vi "Motion Profile Tester.vi"() -> ()   [LabVIEW 2015]
uses:
  <vilib>/Rock Robotics/WPI/CAN/TalonSRX/WPI_CANTalonSRX_APIFeedbackSelect.ctl
  <vilib>/Rock Robotics/WPI/CAN/TalonSRX/WPI_CANTalonSRX_MotionProfileTrajectoryPt.ctl
  <vilib>/Rock Robotics/WPI/CAN/TalonSRX/WPI_CANTalonSRX_APIControlMode.ctl
  <vilib>/Rock Robotics/WPI/MotorControl/WPI_MotorControlOpenCANTalonSRX.vi
panel:
  in  "Slave Motor Inverts":bool[](array[boolean])
  in  "Motor ID":dbl
  in  "Slave Motor IDs":dbl[](array[numeric])
  out "Current State":T1(ring)
  in  "Invert Motor":bool=TRUE
  in  "Execute Motion Profile using only Feedfoward":bool
  in  "Soft Limits (rotations)":T2={"Forward Limit Position"=10000.0, "Reverse Limit Position (should be less than foward limit position)"=-10000.0}
  in  "Reverse Soft Limit Enable":bool
  in  "Forward Soft Limit Enable":bool
  in  "Reverse Feedback Sensor":bool
  in  "Feedback Reference":T3=enum."CTR Magnetic Enc (Absolute)"
  in  "PID Values":T4={"P"=0.21, "I"=0.0021, "D"=3.0, "F"=0.12, "I Zone"=1200.0}
  out "error out":errorcluster
  out "Motor Values while Running Profile":cluster{dbl[], dbl[]}[](graph)
  out "Applied Throttle while Running Profile":cluster{dbl[], dbl[]}(graph)
  in  "Run at 100% Power and Graph":bool
  in  "Abort":bool
  in  "Generate, Load, and Run Profile":bool
  in  "Run Profile":bool
  in  "Load Profile":bool
  in  "Generate Profile and Clear Points":bool
  out "Generated Profile":cluster{dbl[], dbl[]}[](graph)
  in  "Mode":T1(ring)
  in  "Motion Profile Control Frame Rate":dbl=10.0
  in  "Rotations to Travel":dbl
  in  "Max Jerk (rotations/sec^3)":dbl
  in  "Max Acceleration (rotations/sec^2)":dbl
  in  "Max Speed (rotations/sec)":dbl
  # "Basic Motor Configuration Settings"
  # "Motion Profile Settings"
  # "If applied throttle exceeds about .95 at any point in the execution of the profile either max speed acceleration, or jerk must be lowered (or PIDF should be adjusted). If it goes below .8 except at the very beginning or end either max speed, acceleration, or jerk  could be increased. (These numbers are for profiles which are supposed to be completed as quickly as possible. In contexts where the priority is on other things such as reducing the amount of force or jerk acting on a gearbox other metrics must be used.)"
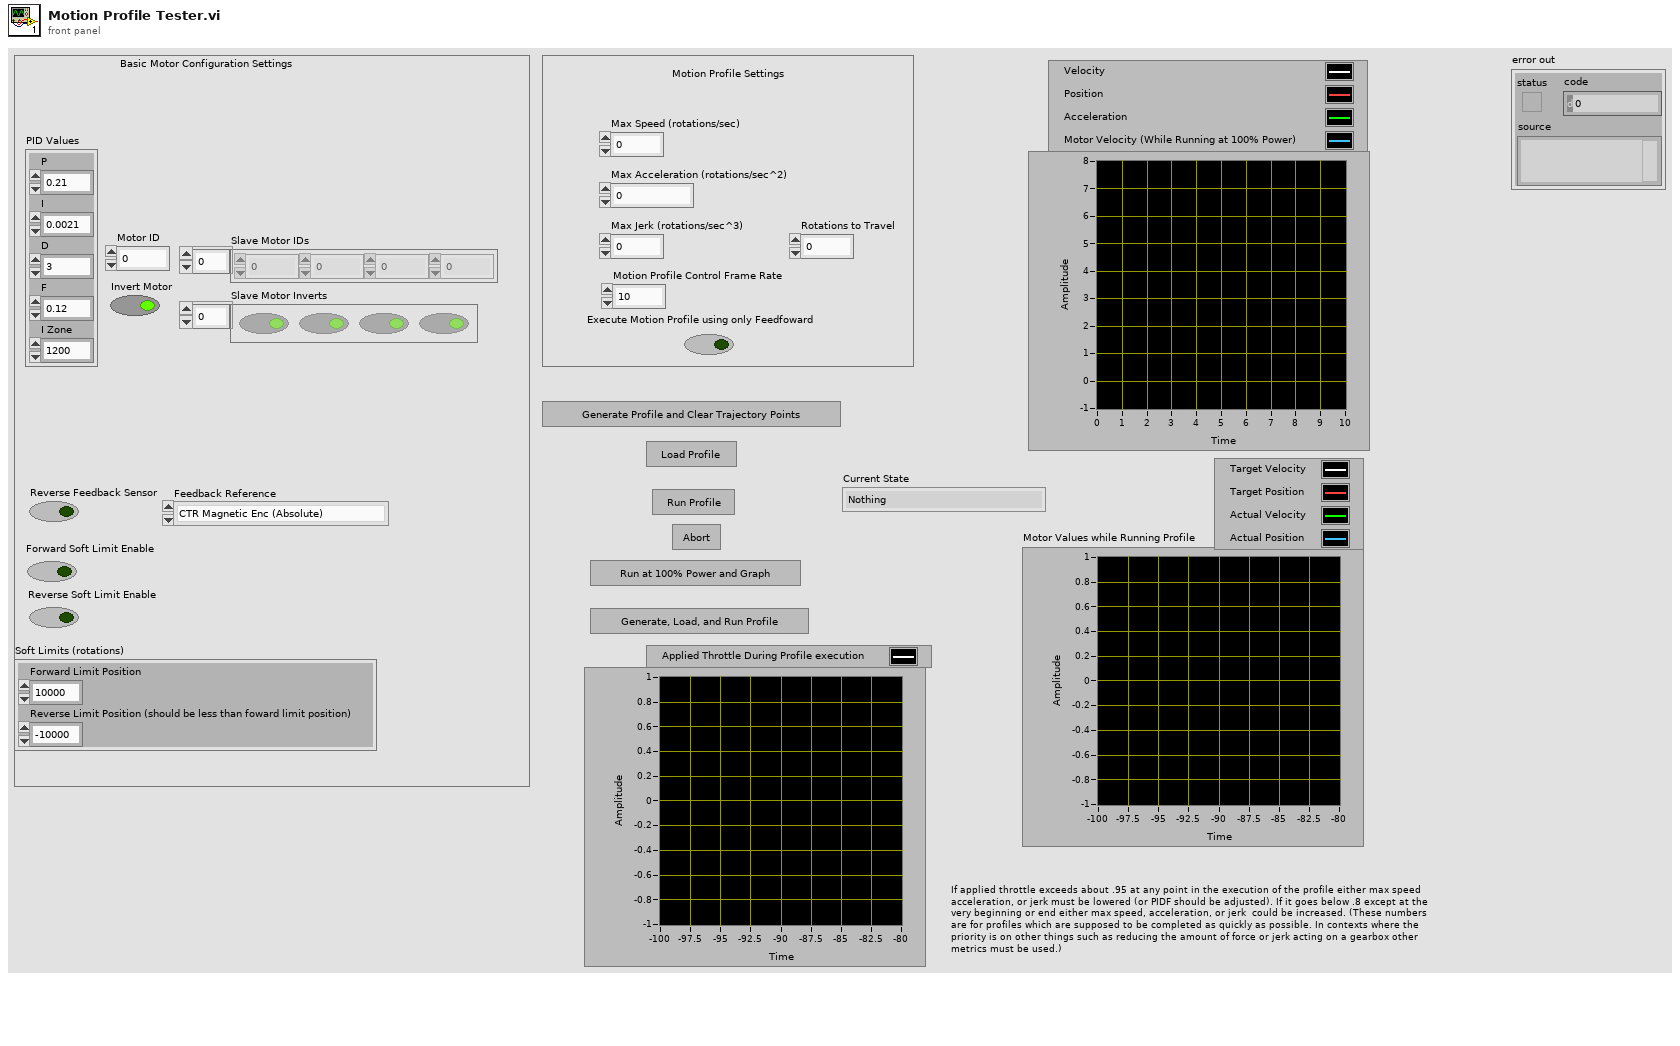
[diagram p1: front panel]
types:
  T1 = enum16{"Nothing", "Generate Profile and Clear", "Load Data to Motor", "Run Profile", "Run at 100% power and log"}
  T2 = cluster{"Forward Limit Position":dbl, "Reverse Limit Position (should be less than foward limit position)":dbl}
  T3 = typedef "WPI_CANTalonSRX_APIFeedbackSelect.ctl" = enum16{"Digital Quadrature Encoder", "Analog Potentiometer", "Analog Encoder", "Count on Quad-A (Rising-Edge)", "Count on Quad-A (Falling-Edge)", "CTR Magnetic Enc (Absolute)", "CTR Magnetic Enc (Relative)", "Pulse Width"}
  T4 = cluster{"P":dbl, "I":dbl, "D":dbl, "F":dbl, "I Zone":dbl}
  T5 = typedef "WPI_CANTalonSRX_APIControlMode.ctl" = enum8{"Percent VBus", "Speed", "Position", "Slave", "Unchanged / Invalid", "Voltage Compensation", "Current", "Motion Profile"}
  T6 = typedef "WPI_MotorControlDeviceRef.ctl" = cluster{"DeviceStatus":errorcluster, "Type":T7, "PWM":cluster{"PWM Channel":T8, "DeadBand":T9}, "CAN":cluster{"Device Number":u8, "Control Mode":T10, "Semaphore":T11, "Max Vout":dbl, "TalonSRX Control Mode":T5}, "Invert":bool}
  T7 = typedef "WPI_MotorControlType.ctl" = enum16{"PWM", "CAN", "CANTalonSRX"}
  T8 = typedef "FPGA_DIOPWMChannel.ctl" = enum8{"PWM 0", "PWM 1", "PWM 2", "PWM 3", "PWM 4", "PWM 5", "PWM 6", "PWM 7", "PWM 8", "PWM 9", "PWM MXP 0", "PWM MXP 1", "PWM MXP 2", "PWM MXP 3", "PWM MXP 4", "PWM MXP 5", "PWM MXP 6", "PWM MXP 7", "PWM MXP 8", "PWM MXP 9", "Invalid"}
  T9 = typedef "WPI_PWMDeadband.ctl" = cluster{"Name":string, "maxPositivePwm":i32, "minPositivePwm":i32, "centerPwm":i32, "maxNegativePwm":i32, "minNegativePwm":i32, "angularRange":u16}
  T10 = typedef "WPI_CANJaguar_ControlMode.ctl" = enum8{"Percent VBus", "Current", "Speed", "Position", "Voltage"}
  T11 = typedef "Semaphore RefNum" = refnum<k1>
  T12 = typedef "WPI_CANTalonSRX_MotionProfileTrajectoryPt.ctl" = cluster{"Duration Ms":u8, "Velocity":dbl, "Position":dbl, "Profile Slot Select":u8, "Is Last":bool, "Velocity Only":bool, "Zero Position":bool, "Compress Code":u8, "Same Velocity":i32, "Delta Position":i32, "Count":u8}
  T13 = enum16{"Nothing", "Generate Profile and Clear", "Load Data to Motor", "Run Profile"}
  T14 = enum16{"Nothing", "Generate Profile and Clear", "Load Data to Motor", "Run Profile", "Run at 100% power and log"}[]
  T15 = typedef "WPI_CANTalonSRX_GlobalStatus.ctl" = cluster{"Applied Throttle":dbl, "Module Enabled":bool, "CAN Error":errorcluster, "Closed Loop Error":dbl, "Forward Limit Switch Closed":bool, "Reverse Limit Switch Closed":bool, "Sensor Position":dbl, "Sensor Velocity":dbl, "Current":dbl, "Sticky Fault - Over Temp":bool, "Sticky Fault - Under Voltage":bool, "Sticky Fault - Forward Limit":bool, "Sticky Fault - Reverse Limit":bool, "Sticky Fault - Forward Soft Limit":bool, "Sticky Fault - Reverse Soft Limit":bool, "Brake is Enabled":bool, "Encoder Position":dbl, "Encoder Velocity":dbl, "Encoder Index Count":dbl, "Encoder A Pin State":bool, "Encoder B Pin State":bool, "Encoder Index Pin State":bool, "Analog In":dbl, "Analog In Velocity":dbl, "Temperature (C)":dbl, "Battery Voltage":dbl, "Control 5 Is Supported":bool, "Current Profile Slot Select":dbl, "Pos Div 8":bool, "Vel Div 4":bool, "Pulse Width Position":i32, "Pulse Width Velocity":i32, "Pulse Width Rise To Rise (us)":i32, "Pulse Width Rise To Fall (us)":i32, "Mot Prof Active Is Under Run":bool, "Mot Prof Active Has Under Run":bool, "Mot Prof Active Is Last":bool, "Mot Prof Active Velocity Only":bool, "Mot Prof Active Is Valid":bool, "Mot Prof Buffer Is Full":bool, "Mot Prof Active Profile Slot Select":i32, "Mot Prof NextID":i32, "Mot Prof Count":i32, "Mot Prof Active Velocity":dbl, "Mot Prof Active Position":dbl, "Mot Prof Output Enable":i32}
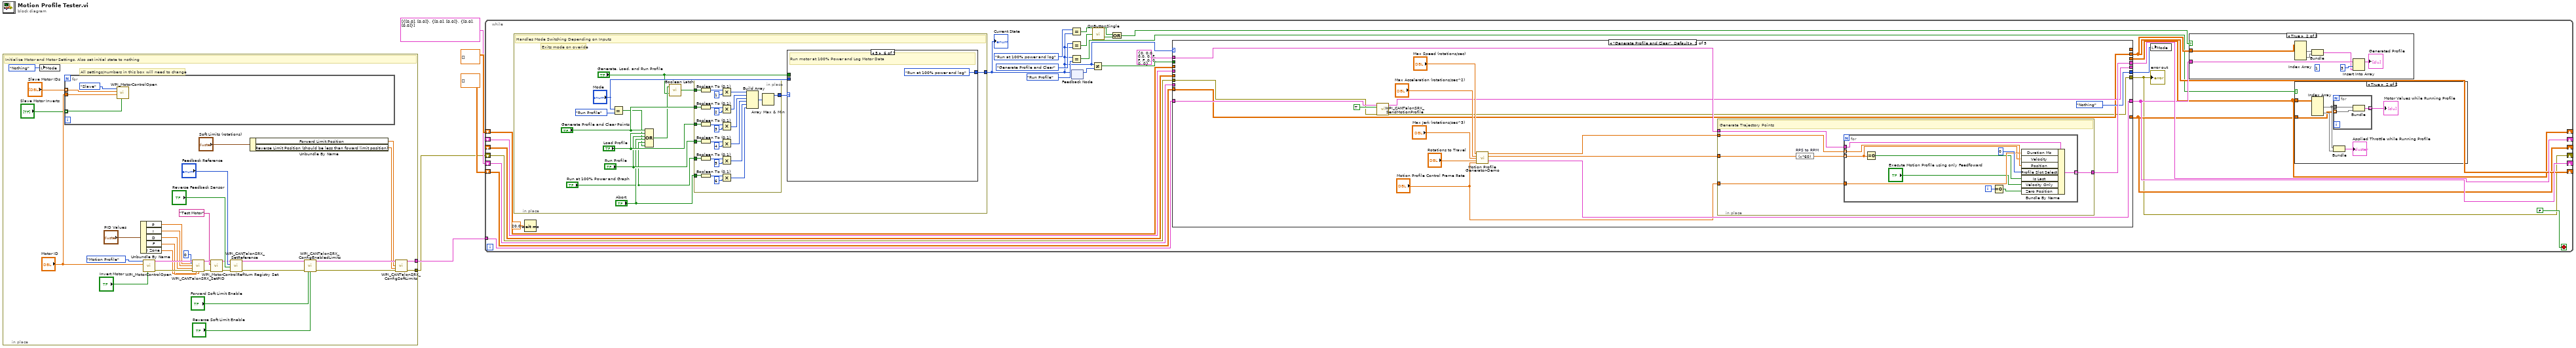
[diagram p0: block diagram]
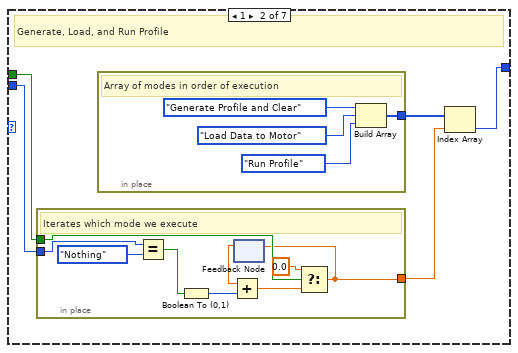
[diagram p5: hidden frame]
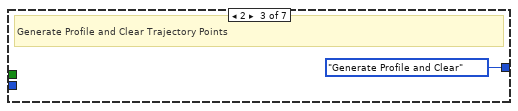
[diagram p6: hidden frame]
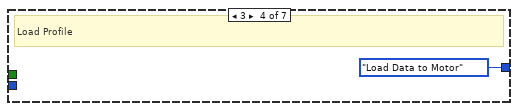
[diagram p7: hidden frame]
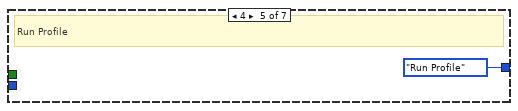
[diagram p8: hidden frame]
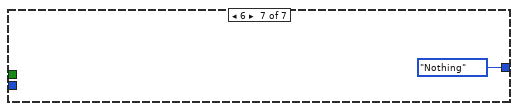
[diagram p9: hidden frame]
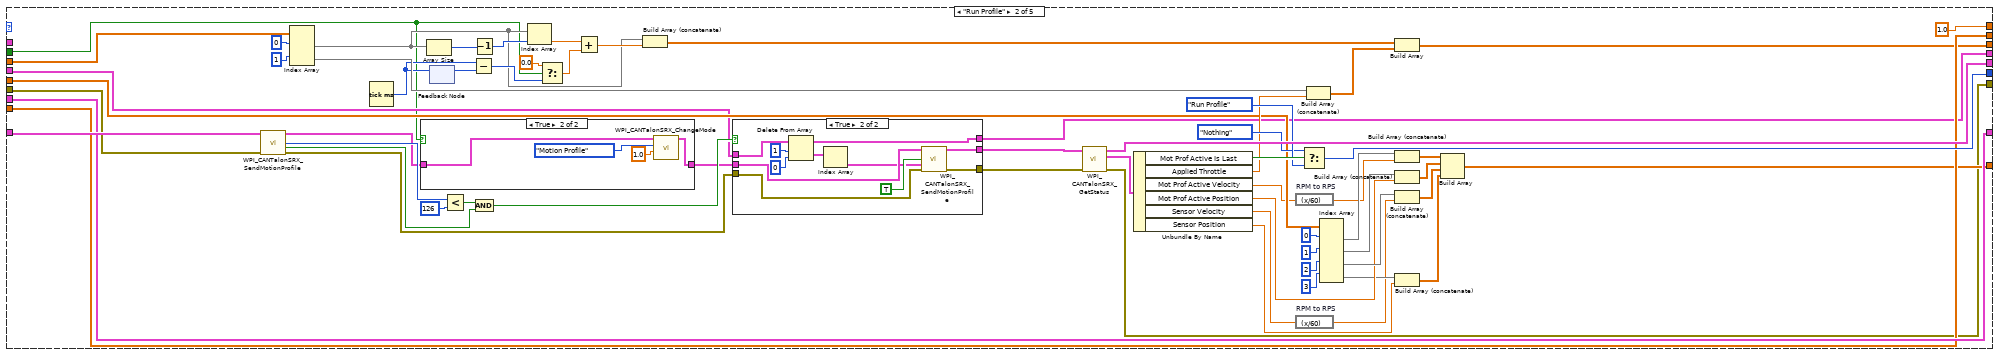
[diagram p10: hidden frame]
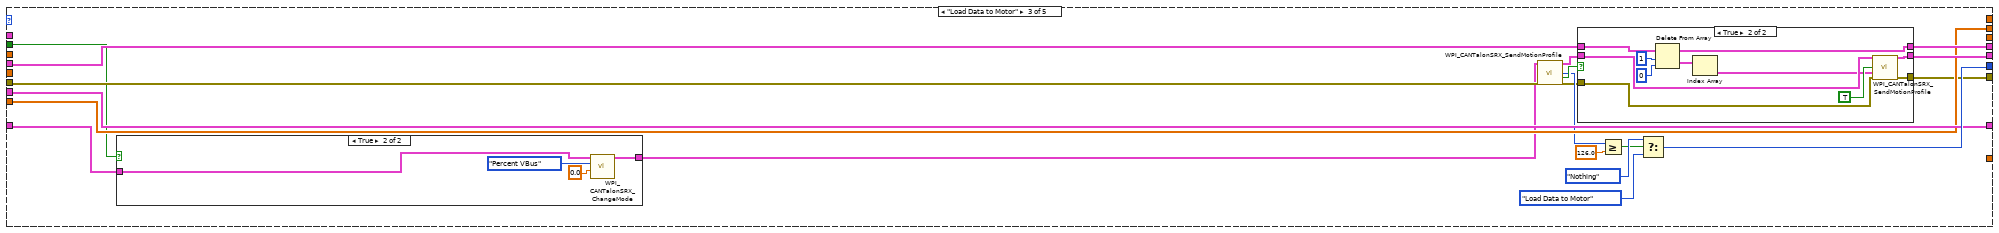
[diagram p13: hidden frame]
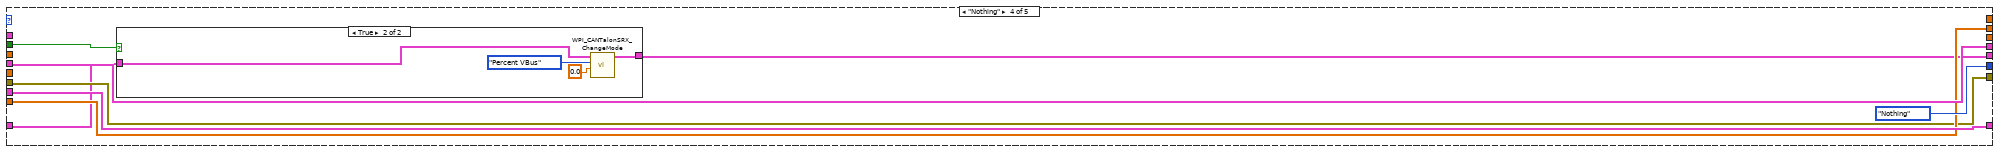
[diagram p16: hidden frame]
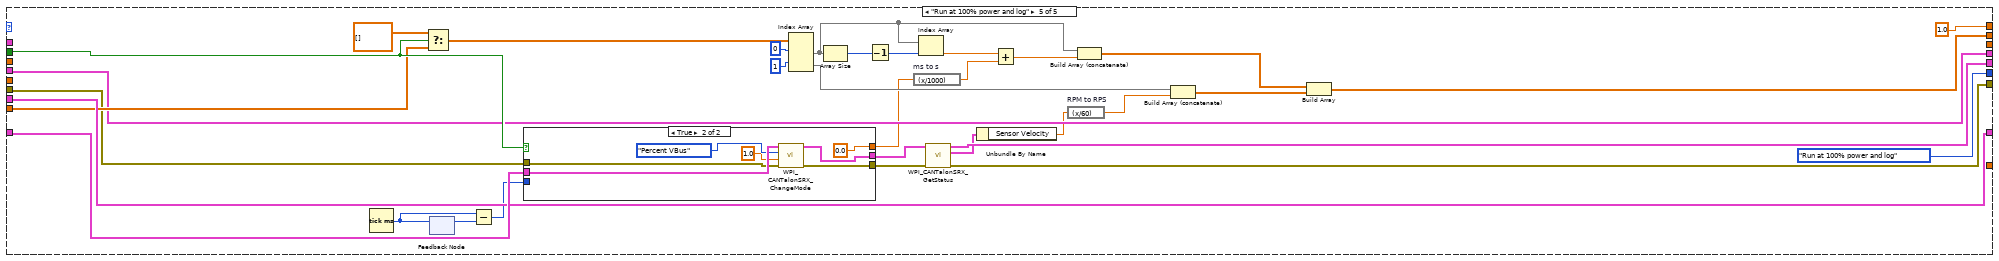
[diagram p18: hidden frame]
diagram:
  n1 = in-place {
    in-place-border: [w33] -> w5
    in-place-border: [w20] -> w1
    # "All settings/numbers in this box will need to change"
    # "Initialize Motor and Motor Settings. Also set initial state to nothing"
    n2 = local write "Mode"(T1."Nothing" ("Mode")) -> ()
    n3 = for {
      tunnel: "Motor ID" -> [w42]
      tunnel: "Slave Motor IDs" -> [w41] mode=indexing
      tunnel: "Slave Motor Inverts" -> [w39] mode=indexing
      n4 = call-poly <vilib>:"WPI_MotorControlOpen.vi"("Invert"=w39, "Master Device Number"=w42, "Device Number"=w41, "Control Mode"=WPI_CANTalonSRX_APIControlMode."Slave") -> ()  [unwired: 6 in, 2 out]
    }
    n5 = Unbundle By Name("PID Values") -> ("P"=w13:dbl, "I"=w12:dbl, "D"=w11:dbl, "F"=w10:dbl, "I Zone"=w9:dbl)
    n6 = call-poly <vilib>:"WPI_MotorControlOpen.vi"("Invert"="Invert Motor", "Device Number"="Motor ID", "Control Mode"=WPI_CANTalonSRX_APIControlMode."Motion Profile") -> ("error out"=w36:errorcluster, "MotorControlDeviceRef"=w37:T6)  [unwired: 7 in]
    n7 = call <vilib>:"WPI_CANTalonSRX_SetPID.vi"("CAN Talon SRX Ref"=w37, "Parameter Slot"=u8 0, "P"=w13, "I"=w12, "D"=w11, "error in (no error)"=w36, "F"=w10, "I Zone"=w9) -> ("CAN Talon SRX Ref"=w28:T6, "error out"=w26:errorcluster)  [unwired: 6 in]
    n8 = call <vilib>:"WPI_MotorControlRefNum Registry Set.vi"("error in (no error)"=w26, "refnum name"="Test Motor", "MotorControlDevRef"=w28) -> ("error out"=w25:errorcluster, "MotorControlDevRef"=w27:T6)  [unwired: 7 in]
    n9 = call <vilib>:"WPI_CANTalonSRX_SetReference.vi"("error in (no error)"=w25, "Reverse Feedback Sensor"="Reverse Feedback Sensor", "Feedback Reference"="Feedback Reference", "CAN Talon SRX Ref"=w27) -> ("error out"=w22:errorcluster, "CAN Talon SRX Ref"=w23:T6)  [unwired: 6 in]
    n10 = Unbundle By Name("Soft Limits (rotations)") -> ("Forward Limit Position"=w16:dbl, "Reverse Limit Position (should be less than foward limit position)"=w15:dbl)
    n11 = call <vilib>:"WPI_CANTalonSRX_ConfigEnabledLimits.vi"("CAN Talon SRX Ref"=w23, "error in (no error)"=w22, "Forward Soft Limit Enable"="Forward Soft Limit Enable", "Reverse Soft Limit Enable"="Reverse Soft Limit Enable") -> ("CAN Talon SRX Ref"=w31:T6, "error out"=w32:errorcluster)  [unwired: 10 in]
    n12 = call <vilib>:"WPI_CANTalonSRX_ConfigSoftLimits.vi"("CAN Talon SRX Ref"=w31, "Forward Limit Position"=w16, "Reverse Limit Position"=w15, "error in (no error)"=w32) -> ("CAN Talon SRX Ref"=w33:T6, "error out"=w20:errorcluster)  [unwired: 10 in]
  }
  n13 = while {
    tunnel: w5 -> [w70]
    shift-right: [w68] -> _
    shift-left: _ -> [w65]
    shift-right: [w59] -> _
    shift-left: cluster{dbl[], dbl[]}[] [{[0.0], [0.0]}, {[0.0], [0.0]}, {[0.0], [0.0]}] ("XY Graph") -> [w61]
    shift-right: [w58] -> _
    shift-left: dbl[][] [] -> [w60]
    shift-right: [w50] -> _
    shift-left: dbl[][] [] -> [w53]
    shift-right: [w48] -> _
    shift-left: _ -> [w49]
    shift-right: [w43] -> _
    shift-left: w1 -> [w44]
    stop <- FALSE stop-if-true
    n14 = in-place {
      in-place-border: [w98] -> w47
      # "Exits mode on overide"
      # "Handles Mode Switching Depending on Inputs"
      n15 = Equal?(x="Mode", y=T13."Run Profile") -> (x = y?=w89:bool)
      n16 = Compound Arithmetic op=OR("Generate Profile and Clear Points", "Load Profile", "Run Profile", "Abort", "Run at 100% Power and Graph", w89) -> (w88:bool)
      n17 = call "Boolean Latch.vi"("Input"="Generate, Load, and Run Profile", "Reset"=w88) -> ("Output"=w95:bool)
      n18 = in-place {
        in-place-border: "Generate Profile and Clear Points" -> [w125]
        in-place-border: "Load Profile" -> [w120]
        in-place-border: w95 -> [w118]
        in-place-border: "Run Profile" -> [w116]
        in-place-border: [w114] -> w96
        in-place-border: "Abort" -> [w105]
        in-place-border: "Run at 100% Power and Graph" -> [w102]
        n19 = Boolean To (0,1)(Boolean=w118) -> (0, 1=w112:i16)
        n20 = Boolean To (0,1)(Boolean=w125) -> (0, 1=w124:i16)
        n21 = Boolean To (0,1)(Boolean=w120) -> (0, 1=w122:i16)
        n22 = Boolean To (0,1)(Boolean=w116) -> (0, 1=w113:i16)
        n23 = Boolean To (0,1)(Boolean=w102) -> (0, 1=w101:i16)
        n24 = Boolean To (0,1)(Boolean=w105) -> (0, 1=w104:i16)
        n25 = Multiply(x=w112, y=i16 1) -> (x*y=w109:i16)
        n26 = Multiply(x=w124, y=i16 2) -> (x*y=w108:i16)
        n27 = Multiply(x=w122, y=i16 3) -> (x*y=w107:i16)
        n28 = Multiply(x=w113, y=i16 4) -> (x*y=w106:i16)
        n29 = Multiply(x=w101, y=i16 5) -> (x*y=w100:i16)
        n30 = Multiply(x=w104, y=i16 6) -> (x*y=w103:i16)
        n31 = Build Array(w109, w108, w107, w106, w100, w103) -> (w115:i16[])
        n32 = Array Max & Min(array=w115) -> (max value=w114:i16)  [unwired: 3 out]
      }
      n33 = case shown="5" w96 {
        tunnel: [w126 w127 T1."Generate Profile and Clear" ("Mode") T1."Load Data to Motor" ("Mode") T1."Run Profile" ("Mode") T1."Run at 100% power and log" ("Mode") T1."Nothing" ("Mode")] -> w98
        tunnel: "Mode" -> [w126 w131 _ _ _ _ _]
        tunnel: "Generate, Load, and Run Profile" -> [_ w130 _ _ _ _ _]
        frame 0, Default {
          # "Carry last operation"
        }
        frame 1 {
          # "Generate, Load, and Run Profile"
          n34 = in-place {
            in-place-border: w131 -> [w140]
            in-place-border: w130 -> [w135]
            in-place-border: [w132] -> w128
            # "Iterates which mode we execute"
            n35 = Equal?(x=w140, y=T13."Nothing") -> (x = y?=w138:bool)
            n36 = Boolean To (0,1)(Boolean=w138) -> (0, 1=w137:i16)
            n37 = feedback #1() -> (w136:dbl)  [unwired: 1 in]
            n38 = Add(x=w136, y=w137) -> (x+y=w133:dbl)
            n39 = Select(t=0.0, s=w135, f=w133) -> (s? t:f=w132:dbl)
            n40 = feedback-in #1(w132) -> ()
          }
          n41 = in-place {
            in-place-border: [w144] -> w129
            # "Array of modes in order of execution"
            n42 = Build Array(T1."Generate Profile and Clear" ("Mode"), T1."Load Data to Motor" ("Mode"), T1."Run Profile" ("Mode")) -> (w144:T14)
          }
          n43 = Index Array(array=w129, index=w128) -> (element=w127:T1)
        }
        frame 2 {
          # "Generate Profile and Clear Trajectory Points"
        }
        frame 3 {
          # "Load Profile"
        }
        frame 4 {
          # "Run Profile"
        }
        frame 5 {
          # "Run motor at 100% Power and Log Motor Data"
        }
        frame 6 {
        }
      }
    }
    "Current State" <- w47
    n44 = Wait (ms)(milliseconds to wait=20.0) -> ()  [unwired: 1 out]
    n45 = Equal?(x=T1."Run at 100% power and log", y=w47) -> (x = y?=w54:bool)
    n46 = Equal?(x=T1."Generate Profile and Clear", y=w47) -> (x = y?=w57:bool)
    n47 = Equal?(x=w47, y=T1."Run Profile") -> (x = y?=w51:bool)
    n48 = feedback-in #2(w47) -> ()
    n49 = feedback #2() -> (w46:T1)  [unwired: 1 in]
    n50 = Not Equal?(x=w47, y=w46) -> (x != y?=w45:bool)
    n51 = call "OnButtonSingle.vi"("Input"=w57) -> ("Released"=w56:bool)  [unwired: 1 out]
    n52 = Or(x=w54, y=w56) -> (x .or. y?=w55:bool)
    n53 = case shown="\"Generate Profile and Clear\", Default" w47 {
      tunnel: w70 -> [w162 w244 w267 w305 w348]
      tunnel: T12 {"Duration Ms"=0, "Velocity"=0.0, "Position"=0.0, "Profile Slot Select"=0, "Is Last"=FALSE, "Velocity Only"=FALSE, "Zero Position"=FALSE, "Compress Code"=0, "Same Velocity"=0, "Delta Position"=0, "Count"=0} ("New Point") -> [w161 _ _ _ _]
      tunnel: [w158 w191 w281 w310 w321] -> w68
      tunnel: [T1."Nothing" ("Mode") w241 w279 T1."Nothing" ("Mode") T1."Run at 100% power and log" ("Mode")] -> w66
      tunnel: w65 -> [_ w192 w283 w310 w321]
      tunnel: [w157 w243 w278 w304 w344] -> _
      tunnel: [_ 1.0 _ _ 1.0] -> _
      tunnel: w45 -> [_ w185 w265 w303 w335]
      tunnel: [w154 w236 w274 w307 w337] -> w58
      tunnel: [w155 w237 w275 w308 w343] -> w59
      tunnel: w61 -> [_ w237 w275 w308 w343]
      tunnel: w60 -> [w154 w236 w274 w307 w334]
      tunnel: w53 -> [_ w186 _ _ _]
      tunnel: [_ w232 _ _ _] -> w50
      tunnel: w49 -> [_ w225 _ _ _]
      tunnel: [_ w212 _ _ _] -> w48
      tunnel: w44 -> [w151 w190 w270 w306 w319]
      tunnel: [w150 w187 w268 w306 w317] -> w43
      frame "Generate Profile and Clear", Default {
        n54 = call <vilib>:"WPI_CANTalonSRX_SendMotionProfile.vi"("CAN Talon SRX Ref"=w162, "Clear"=TRUE, "error in"=w151) -> ("CAN Talon SRX Ref Out"=w157:T6, "error out"=w150:errorcluster)  [unwired: 9 in, 2 out]
        n55 = call "Motion Profile Generator-Demo.vi"("Max Speed (rotations/sec)"="Max Speed (rotations/sec)", "Max Acceleration (rotations/sec^2)"="Max Acceleration (rotations/sec^2)", "Max Jerk (rotations/sec^3)"="Max Jerk (rotations/sec^3)", "Rotations to Travel"="Rotations to Travel", "Motion Profile Control Frame Rate"="Motion Profile Control Frame Rate") -> ("Position rotations"=w159:dbl[], "velocity rotations/sec"=w160:dbl[], "XY Graph"=w155:cluster{dbl[], dbl[]}[])  [unwired: 7 in, 1 out]
        n56 = in-place {
          in-place-border: w161 -> [w172]
          in-place-border: w160 -> [w168]
          in-place-border: w159 -> [w171]
          in-place-border: "Motion Profile Control Frame Rate" -> [w170]
          in-place-border: [w169] -> w158
          # "Generate Trajectory Points"
          n57 = expression code="(x*60)" "RPS to RPM"(w168) -> (w167:dbl[])
          n58 = for {
            tunnel: w172 -> [w182]
            tunnel: w167 -> [w178] mode=indexing
            tunnel: w171 -> [w180] mode=indexing
            tunnel: w170 -> [w179]
            tunnel: [w173] -> w169 mode=indexing
            i -> [w175]
            n59 = Equal To 0?(x=w178) -> (x = 0?=w177:bool)
            n60 = Equal To 0?(x=w175) -> (x = 0?=w174:bool)
            n61 = Bundle By Name(cluster=w182, "Duration Ms"=w179, "Velocity"=w178, "Position"=w180, "Profile Slot Select"=u8 0, "Is Last"=w177, "Velocity Only"="Execute Motion Profile using only Feedfoward", "Zero Position"=w174) -> (w173:T12)
          }
        }
      }
      frame "Run Profile" {
        n62 = call <vilib>:"WPI_CANTalonSRX_SendMotionProfile.vi"("CAN Talon SRX Ref"=w244, "error in"=w190) -> ("CAN Talon SRX Ref Out"=w184:T6, "Count"=w198:u32, "Ready For Next"=w195:bool, "error out"=w189:errorcluster)  [unwired: 10 in]
        n63 = Index Array(array=w186, index (row) #1=0 ("index (row)"), index (row) #2=1 ("index (row)")) -> (element #1=w205:dbl[], element #2=w234:dbl[])  [unwired: 2 in]
        n64 = Tick Count (ms)() -> (millisecond timer value=w211:u32)
        n65 = case shown="True" w185 {
          tunnel: w184 -> [w246 w250]
          tunnel: [w246 w249] -> w183
          frame False {
          }
          frame True {
            n66 = call <vilib>:"WPI_CANTalonSRX_ChangeMode.vi"("Output"=1.0, "Control Mode"=WPI_CANTalonSRX_APIControlMode."Motion Profile", "CAN Talon SRX Ref"=w250) -> ("CAN Talon SRX Ref"=w249:T6)  [unwired: 7 in, 1 out]
          }
        }
        n67 = Array Size(array=w205) -> (size(s)=w207:i32)
        n68 = feedback #3() -> (w210:u32)  [unwired: 1 in]
        n69 = feedback-in #3(w211) -> ()
        n70 = Less?(x=w198, y=u32 126) -> (x < y?=w196:bool)
        n71 = Subtract(x=w211, y=w210) -> (x-y=w208:u32)
        n72 = Decrement(x=w207) -> (x-1=w206:i32)
        n73 = And(x=w196, y=w195) -> (x .and. y?=w194:bool)
        n74 = Index Array(array=w205, index=w206) -> (element=w204:dbl)
        n75 = Select(t=0.0, s=w185, f=w208) -> (s? t:f=w203:dbl)
        n76 = Add(x=w204, y=w203) -> (x+y=w233:dbl)
        n77 = Build Array (concatenate)(w205, w233) -> (w231:dbl[])
        n78 = case shown="True" w194 {
          tunnel: w192 -> [w253 w264]
          tunnel: w183 -> [w252 w261]
          tunnel: [w253 w260] -> w191
          tunnel: [w252 w259] -> w193
          tunnel: w189 -> [w251 w255]
          tunnel: [w251 w254] -> w188
          frame False {
          }
          frame True {
            n79 = Delete From Array(array=w264, length=1, index=0) -> (deleted portion=w262:T12[], array with subset deleted=w260:T12[])
            n80 = Index Array(array=w262) -> (element=w256:T12)  [unwired: 1 in]
            n81 = call <vilib>:"WPI_CANTalonSRX_SendMotionProfile.vi"("CAN Talon SRX Ref"=w261, "Push"=TRUE, "New Point"=w256, "error in"=w255) -> ("CAN Talon SRX Ref Out"=w259:T6, "error out"=w254:errorcluster)  [unwired: 8 in, 2 out]
          }
        }
        n82 = call <vilib>:"WPI_CANTalonSRX_GetStatus.vi"("error in (no error)"=w188, "CAN Talon SRX Ref"=w193) -> ("error out"=w187:errorcluster, "Talon SRX Status"=w242:T15, "CAN Talon SRX Ref"=w243:T6)  [unwired: 7 in]
        n83 = Unbundle By Name(w242) -> ("Mot Prof Active Is Last"=w240:bool, "Applied Throttle"=w235:dbl, "Mot Prof Active Velocity"=w202:dbl, "Mot Prof Active Position"=w218:dbl, "Sensor Velocity"=w200:dbl, "Sensor Position"=w216:dbl)
        n84 = expression code="(x/60)" "RPM to RPS"(w202) -> (w201:dbl)
        n85 = expression code="(x/60)" "RPM to RPS"(w200) -> (w199:dbl)
        n86 = Select(t=T1."Nothing" ("Mode"), s=w240, f=T1."Run Profile" ("Mode")) -> (s? t:f=w241:T1)
        n87 = Build Array (concatenate)(w234, w235) -> (w230:dbl[])
        n88 = Index Array(array=w225, index (row) #1=0 ("index (row)"), index (row) #2=1 ("index (row)"), index (row) #3=2 ("index (row)"), index (row) #4=3 ("index (row)")) -> (element #1=w228:dbl[], element #2=w229:dbl[], element #3=w219:dbl[], element #4=w214:dbl[])  [unwired: 4 in]
        n89 = Build Array(w231, w230) -> (w232:dbl[][])
        n90 = Build Array (concatenate)(w228, w201) -> (w227:dbl[])
        n91 = Build Array (concatenate)(w229, w218) -> (w226:dbl[])
        n92 = Build Array (concatenate)(w219, w199) -> (w217:dbl[])
        n93 = Build Array (concatenate)(w214, w216) -> (w213:dbl[])
        n94 = Build Array(w227, w226, w217, w213) -> (w212:dbl[][])
      }
      frame "Load Data to Motor" {
        n95 = case shown="True" w265 {
          tunnel: w267 -> [w284 w288]
          tunnel: [w284 w287] -> w266
          frame False {
          }
          frame True {
            n96 = call <vilib>:"WPI_CANTalonSRX_ChangeMode.vi"("Output"=0.0, "Control Mode"=WPI_CANTalonSRX_APIControlMode."Percent VBus", "CAN Talon SRX Ref"=w288) -> ("CAN Talon SRX Ref"=w287:T6)  [unwired: 7 in, 1 out]
          }
        }
        n97 = call <vilib>:"WPI_CANTalonSRX_SendMotionProfile.vi"("CAN Talon SRX Ref"=w266, "error in"=w270) -> ("CAN Talon SRX Ref Out"=w282:T6, "Count"=w271:u32, "Ready For Next"=w280:bool, "error out"=w269:errorcluster)  [unwired: 10 in]
        n98 = case shown="True" w280 {
          tunnel: w283 -> [w291 w302]
          tunnel: w282 -> [w290 w299]
          tunnel: [w291 w298] -> w281
          tunnel: [w290 w297] -> w278
          tunnel: w269 -> [w289 w293]
          tunnel: [w289 w292] -> w268
          frame False {
          }
          frame True {
            n99 = Delete From Array(array=w302, length=1, index=0) -> (deleted portion=w300:T12[], array with subset deleted=w298:T12[])
            n100 = Index Array(array=w300) -> (element=w294:T12)  [unwired: 1 in]
            n101 = call <vilib>:"WPI_CANTalonSRX_SendMotionProfile.vi"("CAN Talon SRX Ref"=w299, "Push"=TRUE, "New Point"=w294, "error in"=w293) -> ("CAN Talon SRX Ref Out"=w297:T6, "error out"=w292:errorcluster)  [unwired: 8 in, 2 out]
          }
        }
        n102 = Greater Or Equal?(x=w271, y=126.0) -> (x >= y?=w272:bool)
        n103 = Select(t=T1."Nothing" ("Mode"), s=w272, f=T1."Load Data to Motor" ("Mode")) -> (s? t:f=w279:T1)
      }
      frame "Nothing" {
        n104 = case shown="True" w303 {
          tunnel: w305 -> [w311 w315]
          tunnel: [w311 w314] -> w304
          frame False {
          }
          frame True {
            n105 = call <vilib>:"WPI_CANTalonSRX_ChangeMode.vi"("Output"=0.0, "Control Mode"=WPI_CANTalonSRX_APIControlMode."Percent VBus", "CAN Talon SRX Ref"=w315) -> ("CAN Talon SRX Ref"=w314:T6)  [unwired: 7 in, 1 out]
          }
        }
      }
      frame "Run at 100% power and log" {
        n106 = Tick Count (ms)() -> (millisecond timer value=w325:u32)
        n107 = Select(t=dbl[][] [], s=w335, f=w334) -> (s? t:f=w332:dbl[][])
        n108 = feedback #4() -> (w324:u32)  [unwired: 1 in]
        n109 = feedback-in #4(w325) -> ()
        n110 = Subtract(x=w325, y=w324) -> (x-y=w323:u32)
        n111 = case shown="True" w335 {
          tunnel: w348 -> [w351 w358]
          tunnel: [w351 w357] -> w345
          tunnel: [w350 0.0] -> w316
          tunnel: w323 -> [w350 _]
          tunnel: w319 -> [w349 w355]
          tunnel: [w349 w354] -> w318
          frame False {
          }
          frame True {
            n112 = call <vilib>:"WPI_CANTalonSRX_ChangeMode.vi"("error in (no error)"=w355, "Output"=1.0, "Control Mode"=WPI_CANTalonSRX_APIControlMode."Percent VBus", "CAN Talon SRX Ref"=w358) -> ("error out"=w354:errorcluster, "CAN Talon SRX Ref"=w357:T6)  [unwired: 6 in]
          }
        }
        n113 = Index Array(array=w332, index (row) #1=0 ("index (row)"), index (row) #2=1 ("index (row)")) -> (element #1=w328:dbl[], element #2=w340:dbl[])  [unwired: 2 in]
        n114 = Array Size(array=w328) -> (size(s)=w329:i32)
        n115 = Decrement(x=w329) -> (x-1=w327:i32)
        n116 = expression code="(x/1000)" "ms to s"(w316) -> (w331:dbl)
        n117 = Index Array(array=w328, index=w327) -> (element=w326:dbl)
        n118 = call <vilib>:"WPI_CANTalonSRX_GetStatus.vi"("error in (no error)"=w318, "CAN Talon SRX Ref"=w345) -> ("error out"=w317:errorcluster, "Talon SRX Status"=w322:T15, "CAN Talon SRX Ref"=w344:T6)  [unwired: 7 in]
        n119 = Unbundle By Name(w322) -> ("Sensor Velocity"=w320:dbl)
        n120 = Add(x=w326, y=w331) -> (x+y=w330:dbl)
        n121 = expression code="(x/60)" "RPM to RPS"(w320) -> (w336:dbl)
        n122 = Build Array (concatenate)(w328, w330) -> (w339:dbl[])
        n123 = Build Array (concatenate)(w340, w336) -> (w338:dbl[])
        n124 = Build Array(w339, w338) -> (w337:dbl[][])
      }
    }
    "error out" <- w43
    n125 = local write "Mode"(w66) -> ()
    n126 = case shown="True" w55 {
      tunnel: w59 -> [_ w86]
      tunnel: w58 -> [_ w83]
      frame False {
      }
      frame True {
        (unwired) 1 ("index (row)")
        n127 = Index Array(array=w83) -> (element #1=w82:dbl[], element #2=w81:dbl[])  [unwired: 4 in]
        n128 = Bundle(w82, w81) -> (w80:cluster{dbl[], dbl[]})  [unwired: 1 in]
        n129 = Insert Into Array(array=w86, index=3, new element=w80) -> (→"Generated Profile":cluster{dbl[], dbl[]}[])
      }
    }
    n130 = case shown="True" w51 {
      tunnel: w50 -> [_ w76]
      tunnel: w48 -> [_ w71]
      frame False {
      }
      frame True {
        n131 = Index Array(array=w76) -> (element #1=w72:dbl[], element #2=w75:dbl[])  [unwired: 4 in]
        n132 = for {
          tunnel: w72 -> [w79]
          tunnel: w71 -> [w78] mode=indexing
          tunnel: [w77] -> w73 mode=indexing
          n133 = Bundle(w79, w78) -> (w77:cluster{dbl[], dbl[]})  [unwired: 1 in]
        }
        "Motor Values while Running Profile" <- w73
        n134 = Bundle(w72, w75) -> (→"Applied Throttle while Running Profile":cluster{dbl[], dbl[]})  [unwired: 1 in]
      }
    }
  }
